vi "Opdracht_1_LeesEnSteekInArray.vi"(10 "String 2":string) -> (1 "array w/ subset deleted":string[](array[string]))   [LabVIEW 2018]
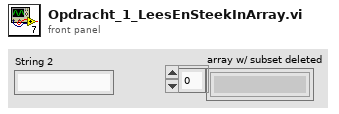
[diagram p1: front panel]
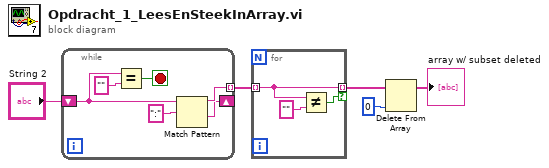
[diagram p0: block diagram]
diagram:
  n1 = while {
    tunnel: [w7] -> w1 mode=indexing
    shift-right: [w6] -> _
    shift-left: "String 2" -> [w8]
    stop <- w9 stop-if-true
    n2 = Equal?(x=w8, y="") -> (x = y?=w9:bool)
    n3 = Match Pattern(string=w8, regular expression=":") -> (before substring=w7:string, after substring=w6:string)  [unwired: 1 in, 2 out]
  }
  n4 = for {
    tunnel: [w14] -> w3 mode=indexing if=w12
    tunnel: w1 -> [w14] mode=indexing
    n5 = Not Equal?(x=w14, y="") -> (x != y?=w12:bool)
  }
  n6 = Delete From Array(array=w3, index=0) -> (array with subset deleted=→"array w/ subset deleted":string[])  [unwired: 1 in, 1 out]
